vi "LoadCustomGlyphs.vi"(7 "tree ref":refnum<vi>, 8 "error in":errorcluster, 11 "glyph directory":path) -> (0 "error out":errorcluster)   [LabVIEW 2013, in "NISE_CEF_TreeControl.lvlib"]
doc: "Adds the glyphs in the folder glyph to the tree control, so nodes can use it."
uses:
  NISE_CEF_TreeControl.lvlib
  Controls/GlyphIndexPair.ctl
  Controls/GlyphIndexPairActions.ctl
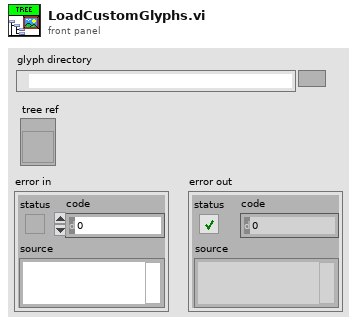
[diagram p1: front panel]
types:
  T1 = typedef "NISE_CEF_TreeControl.lvlib/GlyphIndexPairActions.ctl" = enum16{"Get", "Initialize"}
  T2 = typedef "NISE_CEF_TreeControl.lvlib/GlyphIndexPair.ctl" = cluster{"name":string, "index":i32}
  T3 = typedef "imagedata.ctl" = cluster{"image type":i32, "image depth":i32, "image":u8[], "mask":u8[], "colors":u32[], "Rectangle":cluster{"left":i16, "top":i16, "right":i16, "bottom":i16}}
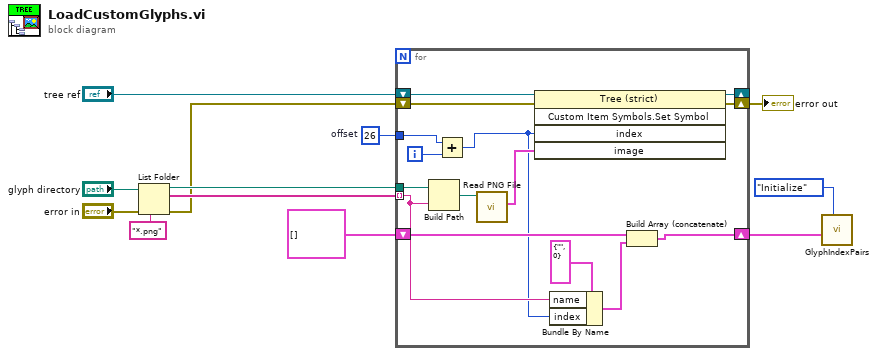
[diagram p0: block diagram]
diagram:
  w6 = 26  # offset
  n1 = List Folder(path="glyph directory", pattern="*.png", error in="error in") -> (path out=w9:path, filenames=w8:string[], error out=w5:errorcluster)  [unwired: 1 in, 1 out]
  n2 = for {
    tunnel: w9 -> [w27]
    tunnel: w8 -> [w18] mode=indexing
    shift-right: [w25] -> _
    shift-left: "tree ref" -> [w26]
    tunnel: w6 -> [w20]
    shift-right: [w14] -> w4
    shift-left: w5 -> [w22]
    shift-right: [w15] -> w2
    shift-left: T2[] [] ("array") -> [w19]
    i -> [w21]
    n3 = Build Path(base path=w27, name or relative path=w18) -> (appended path=w24:path)
    n4 = Add(x=w20, y=w21) -> (x+y=w16:i32)
    n5 = call <vilib>:"Read PNG File.vi"("path to PNG file"=w24) -> ("image data"=w23:T3)  [unwired: 8 in, 2 out]
    n6 = invoke class="Tree (strict)" method="Custom Item Symbols.Set Symbol"(reference=w26, error in=w22, "index"=w16, "image"=w23) -> (reference out=w25:refnum<vi>, error out=w14:errorcluster)  [unwired: 1 in, 3 out]
    n7 = Bundle By Name(cluster=T2 {"name"="", "index"=0} ("glyphIndexPair"), "name"=w18, "index"=w16) -> (w17:T2)
    n8 = Build Array (concatenate)(w19, w17) -> (w15:T2[])
  }
  "error out" <- w4
  n9 = call "GlyphIndexPairs.vi"("enum"=GlyphIndexPairActions."Initialize" ("Enum"), "array"=w2) -> ()  [unwired: 9 in, 1 out]
